vi "Recursive Update Tag.vi"(8 "error in (no error)":errorcluster, 9 "Child Text":string[](array[string]), 10 "Tag":string, 11 "Tag Tree In":refnum<class "Tag Tree.lvclass">) -> (0 "error out":errorcluster, 3 "Tag Tree Out":refnum<class "Tag Tree.lvclass">)   [LabVIEW 2020, in "Tree Helpers.lvlib" / "Tag Tree.lvclass"]
uses:
  Tag Tree.lvclass
  Tag Tree.lvclass/Tag Tree.ctl
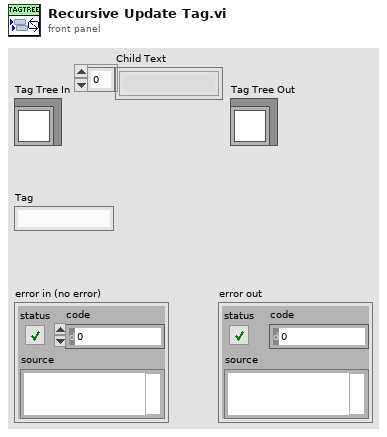
[diagram p1: front panel]
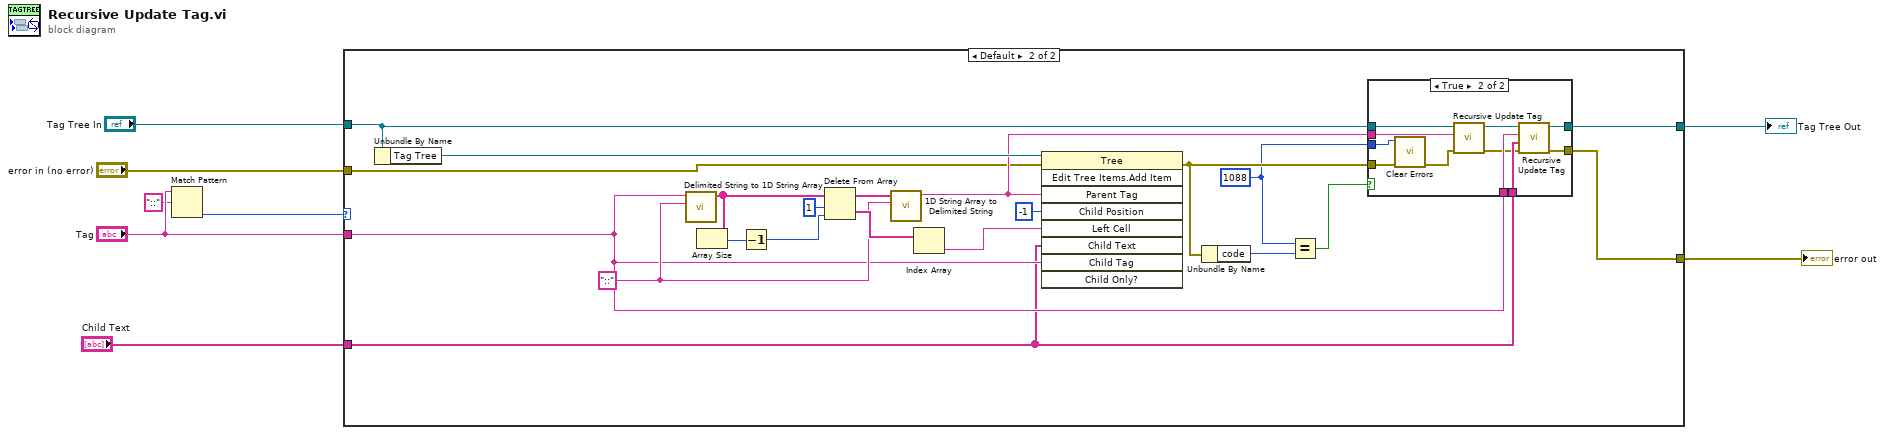
[diagram p0: block diagram]
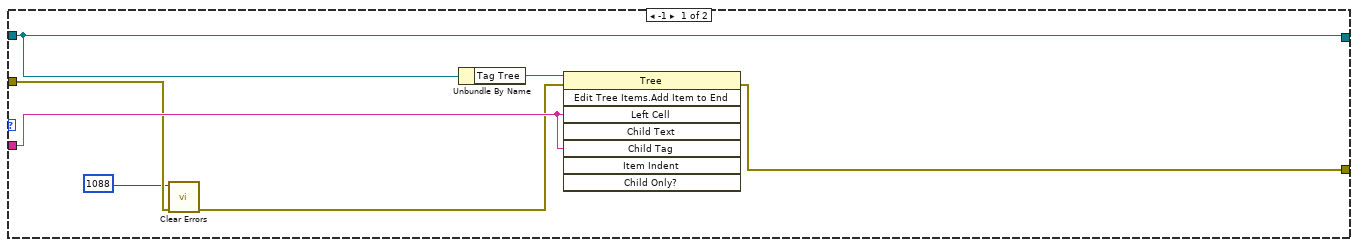
[diagram p2: hidden frame]
diagram:
  n1 = Match Pattern(string="Tag", regular expression="::") -> (offset past match=w2:i32)  [unwired: 1 in, 3 out]
  n2 = case shown="Default" w2 {
    tunnel: "error in (no error)" -> [w11 w18]
    tunnel: [w13 w26] -> w7
    tunnel: "Tag Tree In" -> [w14 w25]
    tunnel: [w14 w24] -> w5
    tunnel: "Tag" -> [w12 w21]
    tunnel: "Child Text" -> [_ w19]
    frame -1 {
      n3 = call <vilib>:"Clear Errors.vi"("error in (no error)"=w11, "specific error code to clear (0: all)"=1088) -> ("error out"=w9:errorcluster)  [unwired: 4 in, 1 out]
      n4 = Unbundle By Name(w14) -> ("Tag Tree"=w15:refnum<vi>)
      n5 = invoke class="Tree" method="Edit Tree Items.Add Item to End"(reference=w15, error in=w9, "Left Cell"=w12, "Child Tag"=w12) -> (error out=w13:errorcluster)  [unwired: 4 in, 7 out]
    }
    frame Default {
      w16 = 1088
      w32 = "::" ("delimiter")
      n6 = Unbundle By Name(w25) -> ("Tag Tree"=w33:refnum<vi>)
      n7 = call <vilib>:"Delimited String to 1D String Array.vi"("delimiter"=w32, "delimited string"=w21) -> ("string array"=w29:string[])  [unwired: 9 in]
      n8 = Array Size(array=w29) -> (size(s)=w27:i32)
      n9 = Decrement(x=w27) -> (x-1=w28:i32)
      n10 = Delete From Array(array=w29, length=1, index=w28) -> (deleted portion=w34:string[], array with subset deleted=w31:string[])
      n11 = call <vilib>:"1D String Array to Delimited String.vi"("delimiter"=w32, "string array"=w31) -> ("delimited string"=w23:string)  [unwired: 9 in]
      n12 = Index Array(array=w34) -> (element=w35:string)  [unwired: 1 in]
      n13 = invoke class="Tree" method="Edit Tree Items.Add Item"(reference=w33, error in=w18, "Parent Tag"=w23, "Child Position"=-1, "Left Cell"=w35, "Child Text"=w19, "Child Tag"=w21) -> (error out=w17:errorcluster)  [unwired: 2 in, 8 out]
      n14 = Unbundle By Name(w17) -> ("code"=w36:i32)
      n15 = Equal?(x=w16, y=w36) -> (x = y?=w22:bool)
      n16 = case shown="True" w22 {
        tunnel: w17 -> [w37 w41]
        tunnel: [w37 w48] -> w26
        tunnel: w25 -> [w38 w44]
        tunnel: [w38 w49] -> w24
        tunnel: w23 -> [_ w42]
        tunnel: w21 -> [_ w47]
        tunnel: w19 -> [_ w46]
        tunnel: w16 -> [_ w40]
        frame False {
        }
        frame True {
          n17 = call <vilib>:"Clear Errors.vi"("error in (no error)"=w41, "specific error code to clear (0: all)"=w40) -> ("error out"=w39:errorcluster)  [unwired: 4 in, 1 out]
          n18 = call "Recursive Update Tag.vi"("error in (no error)"=w39, "Tag"=w42, "Tag Tree In"=w44) -> ("error out"=w43:errorcluster, "Tag Tree Out"=w45:refnum<class "Tag Tree.lvclass">)  [unwired: 7 in]
          n19 = call "Recursive Update Tag.vi"("error in (no error)"=w43, "Child Text"=w46, "Tag"=w47, "Tag Tree In"=w45) -> ("error out"=w48:errorcluster, "Tag Tree Out"=w49:refnum<class "Tag Tree.lvclass">)  [unwired: 6 in]
        }
      }
    }
  }
  "error out" <- w7
  "Tag Tree Out" <- w5
